vi "Insert Subsequence.vi"(6 "Insertion Index":i32=-1, 7 "Parent ID":string, 8 "error in (no error)":errorcluster, 9 "Unique ID":string, 10 "Name":string, 11 "Custom Type Test Executive in":refnum<class "Custom Type Test Executive.lvclass">) -> (0 "error out":errorcluster, 1 "Replaced?":bool, 3 "Custom Type Test Executive out":refnum<class "Custom Type Test Executive.lvclass">, 5 "Unique ID out":string)   [LabVIEW 2017, in "Custom Type Test Executive.lvlib" / "Custom Type Test Executive.lvclass"]
uses:
  <vilib>/gpm_packages/@cs/test-executive/Source/Custom Type Test Executive/Custom Type Test Executive/Custom Type Test Executive.lvclass
  C:/Program Files/National Instruments/LabVIEW 2017/vi.lib/gpm_packages/@cs/test-executive/Source/Test Executive/TestExecutive/Test Executive.lvclass
  <vilib>/gpm_packages/@cs/test-executive/Source/Test Executive/Subsequence/Subsequence.lvclass
  <vilib>/gpm_packages/@cs/data-type-serializer/source/Boolean/Boolean.lvclass/Boolean.ctl
  <vilib>/gpm_packages/@cs/test-executive/Source/Test Executive/TestExecutive/Test Executive.lvclass/Test Executive.ctl
  ee229f31-b495-4c8c-a4be-96e990459e7a.vi
  <vilib>/gpm_packages/@cs/data-type-serializer/source/Boolean/Boolean.lvclass
  <vilib>/gpm_packages/@cs/linked-list/Source/Linked List/ILinkedList/ILinked List.lvclass
  <vilib>/gpm_packages/@cs/linked-list/Source/Linked List/Linked List Ref/Linked List Ref.lvclass
  <vilib>/gpm_packages/@cs/test-executive/Source/Test Executive/TestExecutive/Test Executive.lvclass
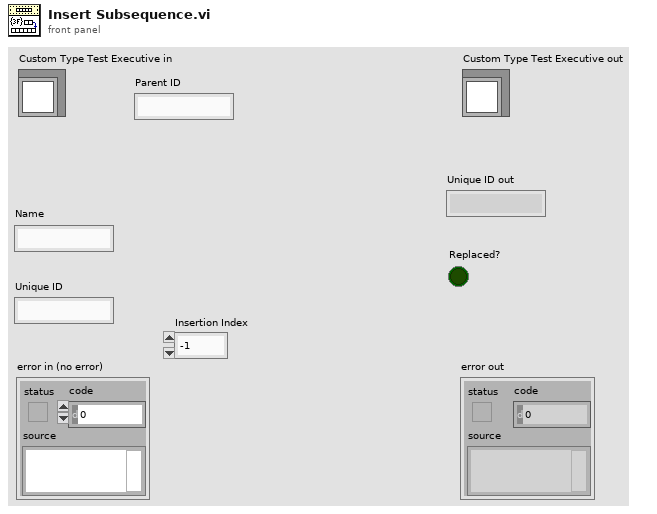
[diagram p1: front panel]
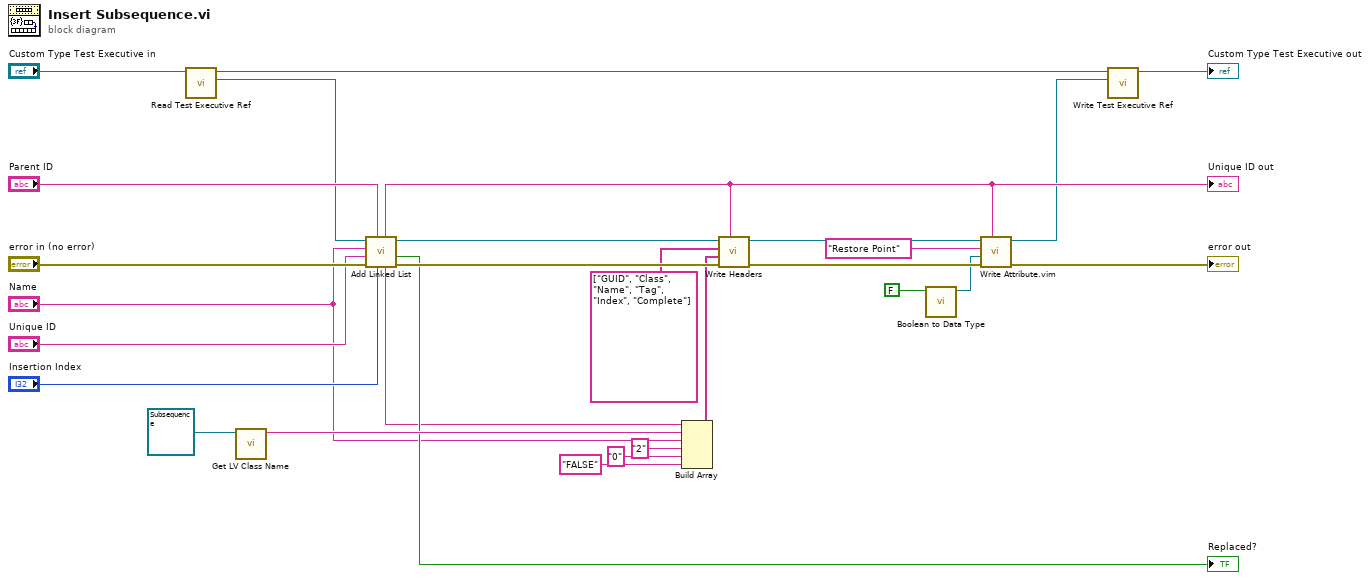
[diagram p0: block diagram]
diagram:
  n1 = call <vilib>:"Read Test Executive Ref.vi"("Test Executive in"="Custom Type Test Executive in") -> ("Test Executive Ref"=w6:refnum<data-value>, "Test Executive out"=w5:refnum<class "Custom Type Test Executive.lvclass">)  [unwired: 9 in]
  n2 = call <vilib>:"Get LV Class Name.vi"("object"=refnum<class "Subsequence.lvclass"> refnum ("Test Executive.lvlib:Subsequence.lvclass")) -> ("class name"=w23:string)  [unwired: 9 in, 1 out]
  n3 = call <vilib>:"Add Linked List.vi"("Insertion Index"="Insertion Index", "Parent ID"="Parent ID", "error in (no error)"="error in (no error)", "Linked List ID"="Unique ID", "Name"="Name", "Linked List Ref"=w6) -> ("error out"=w25:errorcluster, "Replaced?"=→"Replaced?":bool, "Linked List Ref out"=w26:refnum<data-value>, "Linked List ID out"=w8:string)  [unwired: 2 in]
  "Unique ID out" <- w8
  n4 = Build Array(w8, w23, "Name", "2" ("element"), "0" ("element"), "FALSE" ("element")) -> (w21:string[])
  n5 = call <vilib>:"Write Headers.vi"("Linked List ID"=w8, "error in (no error)"=w25, "Header Values"=w21, "Header Names"=string[] ["GUID", "Class", "Name", "Tag", "Index", "Complete"], "Linked List Ref"=w26) -> ("error out"=w18:errorcluster, "Linked List Ref out"=w19:refnum<data-value>)  [unwired: 5 in]
  n6 = call <vilib>:"Boolean to Data Type.vi"("Boolean"=FALSE) -> ("Boolean out"=w1:refnum<class "Boolean.lvclass">)  [unwired: 9 in, 1 out]
  n7 = call "Write Attribute.vim"("Linked List ID"=w8, "error in (no error)"=w18, "Attribute"=w1, "Attribute Name"="Restore Point", "Linked List Ref"=w19) -> ("error out"=→"error out":errorcluster, "Linked List Ref out"=w3:refnum<data-value>)  [unwired: 3 in, 2 out]
  n8 = call <vilib>:"Write Test Executive Ref.vi"("Test Executive Ref"=w3, "Test Executive in"=w5) -> ("Test Executive out"=→"Custom Type Test Executive out":refnum<class "Custom Type Test Executive.lvclass">)  [unwired: 9 in]
